vi "GPOCT_Init.vi"(9 "Dispersion Compensation":T1={"DC_Offset"=1024, "DC_QuadraticA2"=0.0, "DC_QuadrupelA4"=0.0}, 10 "ResamplingVector":dbl[](array[numeric]), 11 "Array":i32[](array[numeric])) -> (0 "error out":errorcluster, 2 "SizeParam":i32[](array[numeric]), 3 "path out":path)   [LabVIEW 2016]
panel:
  in  "path in":path=path "C:/Users/Mikael/Documents/Visual Studio 2015/Projects/GPOCT/x64/Release/GPOCT.dll"
  # "Note: In the SizeParams Array the size of the array\nSizeParams[0]: A-Scan length\nSizeParams[1]: B-Scan length\nSizeParams[2]: Nr of B-Scans\n\nIf DC_Offset is -1, no dispersion correction is applied"
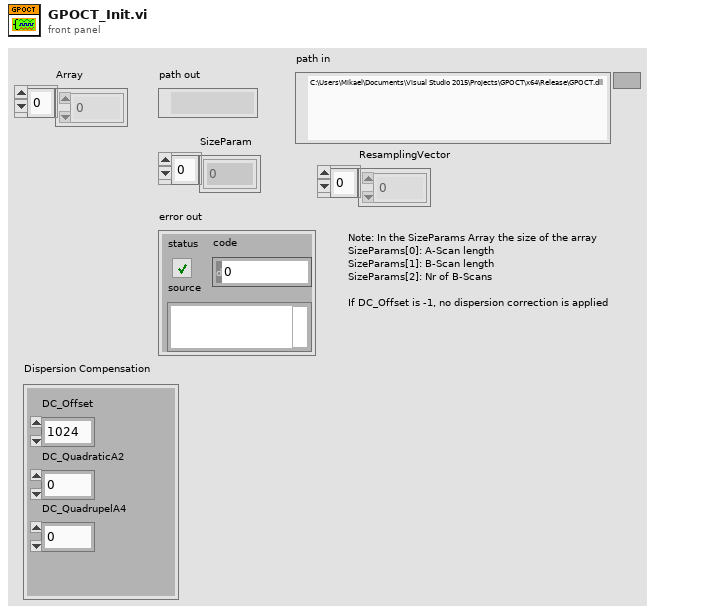
[diagram p1: front panel]
types:
  T1 = cluster{"DC_Offset":i32, "DC_QuadraticA2":dbl, "DC_QuadrupelA4":dbl}
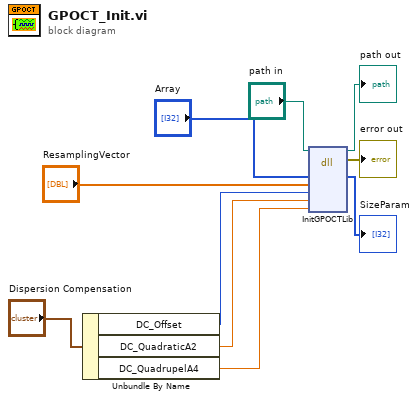
[diagram p0: block diagram]
diagram:
  n1 = Unbundle By Name("Dispersion Compensation") -> ("DC_Offset"=w3:i32, "DC_QuadraticA2"=w2:dbl, "DC_QuadrupelA4"=w1:dbl)
  n2 = dll-call lib="C:/Users/Mikael/Documents/Visual Studio 2015/Projects/GPOCT/x64/Release/GPOCT.dll" fn="InitGPOCTLib"(path in="path in", "SizeParam"="Array", "ResamplingVector"="ResamplingVector", "DC_Offset"=w3, "DC_QuadraticA2"=w2, "DC_QuadrupelA4"=w1) -> (path out=→"path out":path, error out=→"error out":errorcluster, "SizeParam"=→"SizeParam":i32[])  [unwired: 7 in]
